vi "disk_createDiskTemplate.vi"(8 "error in (no error)":errorcluster, 11 "File path":path) -> (0 "error out":errorcluster, 3 "output cluster":T1)   [LabVIEW 2020, in "NI_ExcelFile.lvlib"]
uses:
  <vilib>/express/express shared/NI_ExcelFile/NI_ExcelFile.lvlib
  <vilib>/express/express shared/NI_ExcelFile/Ctrls/disk_TemplateFile.ctl
  <vilib>/express/express shared/NI_ExcelFile/Ctrls/meta_file.ctl
  <vilib>/express/express shared/NI_ExcelFile/Ctrls/meta_Block.ctl
  <vilib>/express/express shared/NI_ExcelFile/Ctrls/meta_BlockType.ctl
  <vilib>/express/express shared/NI_ExcelFile/Ctrls/TemplateEnum.ctl
panel:
  in  "Disk template header":string[](array[string])=["<?xml version=\"1.0\" encoding=\"UTF-8\" standalone=\"yes\"?>\n<Types xmlns=\"http://schemas.openxmlformats.org/package/2006/content-types\">\n  <Default Extension=\"rels\" ContentType=\"application/vnd.openxmlformats-package.relationships+xml\"/>\n  <Override PartName=\"/xl/workbook.xml\" ContentType=\"application/vnd.openxmlformats-officedocument.spreadsheetml.sheet.main+xml\"/>\n  <Override PartName=\"/xl/worksheets/sheet1.xml\" ContentType=\"application/vnd.openxmlformats-officedocument.spreadsheetml.worksheet+xml\"/>\n  <Override PartName=\"/xl/styles.xml\" ContentType=\"application/vnd.openxmlformats-officedocument.spreadsheetml.styles+xml\" />\n  <Override PartName=\"/docProps/app.xml\" ContentType=\"application/vnd.openxmlformats-officedocument.extended-properties+xml\"/>\n  <Override PartName=\"/docProps/core.xml\" ContentType=\"application/vnd.openxmlformats-package.core-properties+xml\"/>\n  <Override PartName =\"/NI/meta\" ContentType = \"application/octet-stream\"/><Override PartName=\"/xl/sharedStrings.xml\" ContentType=\"application/vnd.openxmlformats-officedocument.spreadsheetml.sharedStrings+xml\"/>\n</Types>", "<?xml version=\"1.0\" encoding=\"UTF-8\" standalone=\"yes\"?>\n<Relationships xmlns=\"http://schemas.openxmlformats.org/package/2006/relationships\">\n  <Relationship Id=\"rId3\" Type=\"http://schemas.openxmlformats.org/officeDocument/2006/relationships/extended-properties\" Target=\"docProps/app.xml\"/>\n\t <Relationship Id=\"rId2\" Type=\"http://schemas.openxmlformats.org/package/2006/relationships/metadata/core-properties\" Target=\"docProps/core.xml\"/>\n  <Relationship Id=\"rId1\" Type=\"http://schemas.openxmlformats.org/officeDocument/2006/relationships/officeDocument\" Target=\"xl/workbook.xml\"/>\n</Relationships>", "<?xml version=\"1.0\" encoding=\"UTF-8\" standalone=\"yes\"?>\n<workbook xmlns=\"http://schemas.openxmlformats.org/spreadsheetml/2006/main\" xmlns:r=\"http://schemas.openxmlformats.org/officeDocument/2006/relationships\">\n  <workbookPr date1904=\"true\" />\n  <sheets>\n    <sheet name= \"", "", "<?xml version=\"1.0\" encoding=\"UTF-8\" standalone=\"yes\"?>\n<Relationships xmlns=\"http://schemas.openxmlformats.org/package/2006/relationships\">\n  <Relationship Id=\"rId1\" Target=\"worksheets/sheet1.xml\" Type=\"http://schemas.openxmlformats.org/officeDocument/2006/relationships/worksheet\"/>\n  <Relationship Id=\"rId2\" Target=\"styles.xml\" Type=\"http://schemas.openxmlformats.org/officeDocument/2006/relationships/styles\" /><Relationship Target=\"sharedStrings.xml\" Type=\"http://schemas.openxmlformats.org/officeDocument/2006/relationships/sharedStrings\" Id=\"rId3\"/>\n</Relationships>", "<?xml version=\"1.0\" encoding=\"UTF-8\" standalone=\"yes\"?><worksheet xmlns=\"http://schemas.openxmlformats.org/spreadsheetml/2006/main\" xmlns:r=\"http://schemas.openxmlformats.org/officeDocument/2006/relationships\"><sheetData>", "<?xml version=\"1.0\" encoding=\"UTF-8\" standalone=\"yes\"?>\n<Properties xmlns=\"http://schemas.openxmlformats.org/officeDocument/2006/extended-properties\" xmlns:vt=\"http://schemas.openxmlformats.org/officeDocument/2006/docPropsVTypes\">\n\t<Application>Microsoft Excel</Application>\n\t<DocSecurity>0</DocSecurity>\n\t<ScaleCrop>false</ScaleCrop>\n\t<HeadingPairs>\n\t\t<vt:vector size=\"2\" baseType=\"variant\">\n\t\t\t<vt:variant>\n\t\t\t\t<vt:lpstr>Worksheets</vt:lpstr>\n\t\t\t</vt:variant>\n\t\t\t<vt:variant>\n\t\t\t\t<vt:i4>1</vt:i4>\n\t\t\t</vt:variant>\n\t\t</vt:vector>\n\t</HeadingPairs>\n\t<TitlesOfParts>\n\t\t<vt:vector size=\"1\" baseType=\"lpstr\">\n\t\t\t<vt:lpstr>Sheet1</vt:lpstr>\t\n\t\t</vt:vector>\n\t</TitlesOfParts>\n\t<Company></Company>\n\t<LinksUpToDate>false</LinksUpToDate>\n\t<SharedDoc>false</SharedDoc>\n\t<HyperlinksChanged>false</HyperlinksChanged>\n\t<AppVersion>12.0000</AppVersion>\n</Properties> ", "<?xml version=\"1.0\" encoding=\"UTF-8\" standalone=\"yes\"?>\n<cp:coreProperties xmlns:cp=\"http://schemas.openxmlformats.org/package/2006/metadata/core-properties\" xmlns:dc=\"http://purl.org/dc/elements/1.1/\" xmlns:dcterms=\"http://purl.org/dc/terms/\" xmlns:dcmitype=\"http://purl.org/dc/dcmitype/\" xmlns:xsi=\"http://www.w3.org/2001/XMLSchema-instance\"><dc:creator>", "<?xml version=\"1.0\" encoding=\"UTF-8\" standalone=\"yes\"?><sst xmlns=\"http://schemas.openxmlformats.org/spreadsheetml/2006/main\"><si><t>Inf</t></si><si><t>-Inf</t></si><si><t>#NV</t></si></sst>"]
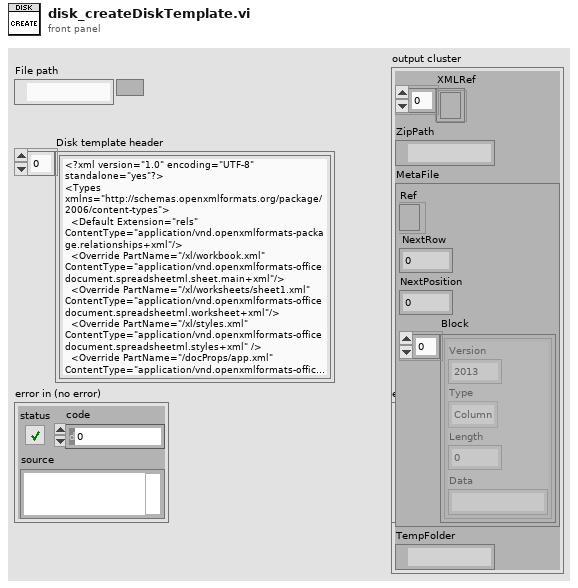
[diagram p1: front panel]
types:
  T1 = typedef "NI_ExcelFile.lvlib/disk_TemplateFile.ctl" = cluster{"XMLRef":refnum<file>[], "ZipPath":path, "MetaFile":T2, "TempFolder":path}
  T2 = typedef "NI_ExcelFile.lvlib/meta_file.ctl" = cluster{"Ref":refnum<file>, "NextRow":i32, "NextPosition":i64, "Block":T3[]}
  T3 = typedef "NI_ExcelFile.lvlib/meta_Block.ctl" = cluster{"Version":u16, "Type":T4, "Length":i32, "Data":string}
  T4 = typedef "NI_ExcelFile.lvlib/meta_BlockType.ctl" = enum16{"NITag", "File", "Column"}
  T5 = typedef "NI_ExcelFile.lvlib/TemplateEnum.ctl" = enum16{"[Content_Types].xml", ".rels", "workbook.xml", "styles.xml", "workbook.xml.rels", "sheet.xml", "app.xml", "core.xml"}
  T6 = enum16{"open", "replace", "create", "open or create", "replace or create", "replace or create with confirmation"}
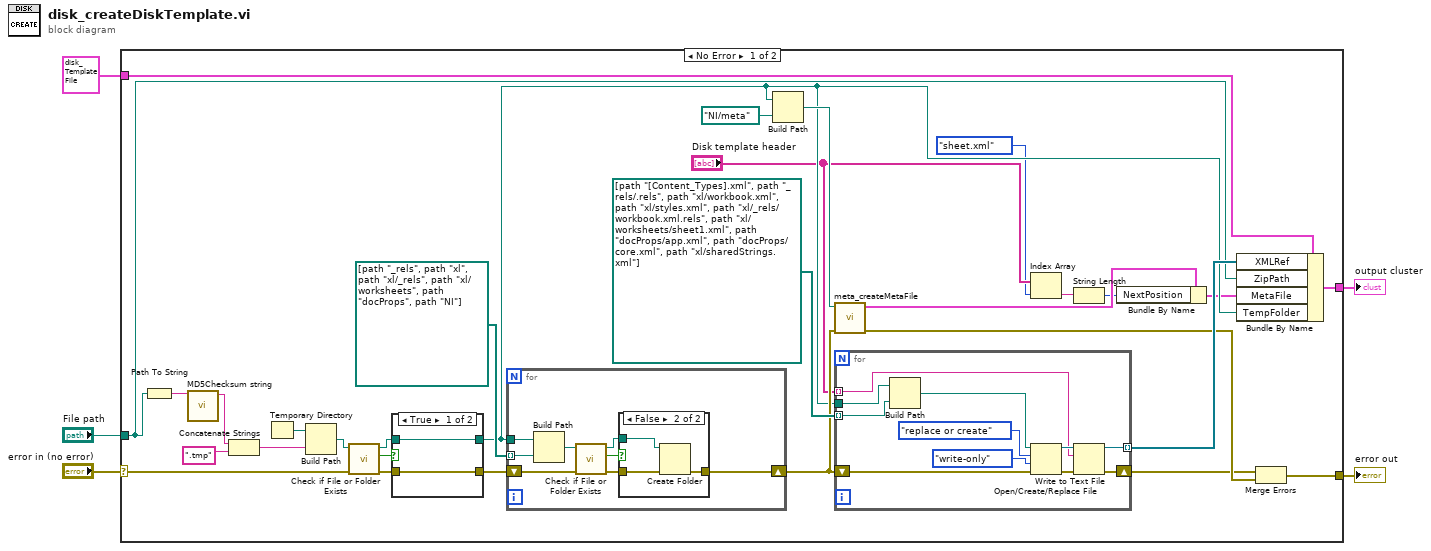
[diagram p0: block diagram]
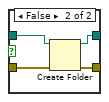
[diagram p2: hidden frame]
diagram:
  n1 = case shown="No Error" "error in (no error)" {
    selector: "error in (no error)" -> [w10 w66]
    tunnel: T1 {"XMLRef"=[refnum, refnum, refnum, refnum, refnum, refnum], "ZipPath"=path "", "MetaFile"={"Ref"=refnum, "NextRow"=0, "NextPosition"=0, "Block"=[]}, "TempFolder"=path ""} ("XLSX file") -> [w34 w65]
    tunnel: [w32 w65] -> w4
    tunnel: "File path" -> [w8 _]
    tunnel: [w20 w66] -> w2
    frame No Error {
      n2 = Path To String(path=w8) -> (string=w7:string)
      n3 = call <vilib>:"MD5Checksum string.vi"("Message String"=w7) -> ("MD5 message-digest"=w6:string)  [unwired: 10 in]
      n4 = Concatenate Strings(w6, ".tmp" ("string")) -> (w12:string)
      n5 = Temporary Directory() -> (w29:path)
      n6 = Build Path(base path=w29, name or relative path=w12) -> (appended path=w25:path)
      n7 = call <vilib>:"Check if File or Folder Exists.vi"("error in (no error)"=w10, "path"=w25) -> ("error out"=w27:errorcluster, "file or folder exists?"=w28:bool, "dup path"=w26:path)  [unwired: 7 in]
      n8 = case shown="True" w28 {
        tunnel: [w37 w41] -> w30
        tunnel: w26 -> [w36 w40]
        tunnel: w27 -> [w37 w39]
        tunnel: [w36 w38] -> w18
        frame True {
        }
        frame False {
          n9 = Create Folder(path (use dialog)=w40, error in=w39) -> (created path=w38:path, error out=w41:errorcluster)  [unwired: 1 in, 1 out]
        }
      }
      n10 = for {
        tunnel: path[] [path "_rels", path "xl", path "xl/_rels", path "xl/worksheets", path "docProps", path "NI"] -> [w47] mode=indexing
        shift-right: [w49] -> w23
        shift-left: w30 -> [w44]
        tunnel: w18 -> [w48]
        n11 = Build Path(base path=w48, name or relative path=w47) -> (appended path=w45:path)
        n12 = call <vilib>:"Check if File or Folder Exists.vi"("error in (no error)"=w44, "path"=w45) -> ("error out"=w43:errorcluster, "file or folder exists?"=w42:bool, "dup path"=w46:path)  [unwired: 7 in]
        n13 = case shown="False" w42 {
          tunnel: [w50 w53] -> w49
          tunnel: w46 -> [_ w52]
          tunnel: w43 -> [w50 w51]
          frame True {
          }
          frame False {
            n14 = Create Folder(path (use dialog)=w52, error in=w51) -> (error out=w53:errorcluster)  [unwired: 1 in, 2 out]
          }
        }
      }
      n15 = Build Path(base path=w18, name or relative path=path "NI/meta") -> (appended path=w24:path)
      n16 = call <vilib>:"meta_createMetaFile.vi"("error in"=w23, "file path"=w24) -> ("error out"=w22:errorcluster, "meta file"=w17:T2)  [unwired: 8 in]
      n17 = for {
        tunnel: path[] [path "[Content_Types].xml", path "_rels/.rels", path "xl/workbook.xml", path "xl/styles.xml", path "xl/_rels/workbook.xml.rels", path "xl/worksheets/sheet1.xml", path "docProps/app.xml", path "docProps/core.xml", path "xl/sharedStrings.xml"] -> [w55] mode=indexing
        shift-right: [w58] -> w21
        shift-left: w23 -> [w57]
        tunnel: "Disk template header" -> [w60] mode=indexing
        tunnel: [w61] -> w33 mode=indexing
        tunnel: w18 -> [w56]
        n18 = Build Path(base path=w56, name or relative path=w55) -> (appended path=w54:path)
        n19 = Open/Create/Replace File(file path (use dialog)=w54, error in=w57, operation (0:open)=T6."replace or create", access (0:read/write)=enum16{"read/write", "read-only", "write-only"}."write-only") -> (refnum out=w62:refnum<file>, error out=w59:errorcluster)  [unwired: 2 in, 1 out]
        n20 = Write to Text File(file (use dialog)=w62, text=w60, error in=w59) -> (refnum out=w61:refnum<file>, error out=w58:errorcluster)  [unwired: 1 in, 1 out]
      }
      n21 = Index Array(array="Disk template header", index=TemplateEnum."sheet.xml" ("Template")) -> (element=w14:string)
      n22 = String Length(string=w14) -> (length=w13:i32)
      n23 = Bundle By Name(cluster=w17, "NextPosition"=w13) -> (w16:T2)
      n24 = Bundle By Name(cluster=w34, "XMLRef"=w33, "ZipPath"=w8, "MetaFile"=w16, "TempFolder"=w18) -> (w32:T1)
      n25 = Merge Errors(w21, w22) -> (w20:errorcluster)
    }
    frame Error {
    }
  }
  "error out" <- w2
  "output cluster" <- w4
